vi "UI_HighEnd.vi"() -> ()   [LabVIEW 2021]
uses:
  Common/LabVIEW GEA2 Toolkit/GEA3/type defs/Data Type.ctl
  Controls/All_Bundled_UI.ctl
  Controls/Cluster leds 3-5.ctl
  D:/Common/LabVIEW GEA2 Toolkit/source/GEA3 DLL Source/GeaCommunication.dll
  Common/LabVIEW GEA2 Toolkit/source/GEA3 DLL Source/GeaCommunication.dll
  Common/LabVIEW GEA2 Toolkit/GEA3/library/GEA2_Toolkit.lvlib
panel:
  in  "Cluster Leds 3-5 2":T1
  in  "All_Bundled_UI":T2
  in  "Knob":dbl(knob) scale=0.0..10.0
  in  "PLANCHA FÁCIL":bool caption="PLANCHA\nFÁCIL"
  in  "LAVADO RÁPIDO":bool caption="LAVADO\nRÁPIDO"
  in  "INICIO PAUSA":bool caption="INICIO\nPAUSA"
  in  "VEL CENTRIF.":bool caption="VEL\nCENTRIF."
  in  "INICIO DIFERIDO":bool caption="INICIO\nDIFERIDO"
  in  "SUPER  ENJUAGUE":bool caption="SUPER \nENJUAGUE"
  in  "TEMP.":bool
  out "ERD Data Out":cluster{"ERD Number":u16, "Data":string}[](array[cluster]) {"ERD Number" format="%.0x"}
  in  "Read ERD List":cluster{"ERD Number":u16, "Data Type":T3}[](array[cluster]) {"ERD Number" format="%.0x"}
  in  "GEA Inputs":cluster{"Source":u8, "Destination":u8}={"Source"=229, "Destination"=192} {"Destination" format="%.0x"; "Source" format="%.0x"}
  in  "Read":bool=TRUE
  in  "Stop Button":bool
  # "70°C"
  # "60°C"
  # "40°C"
  # "30°C"
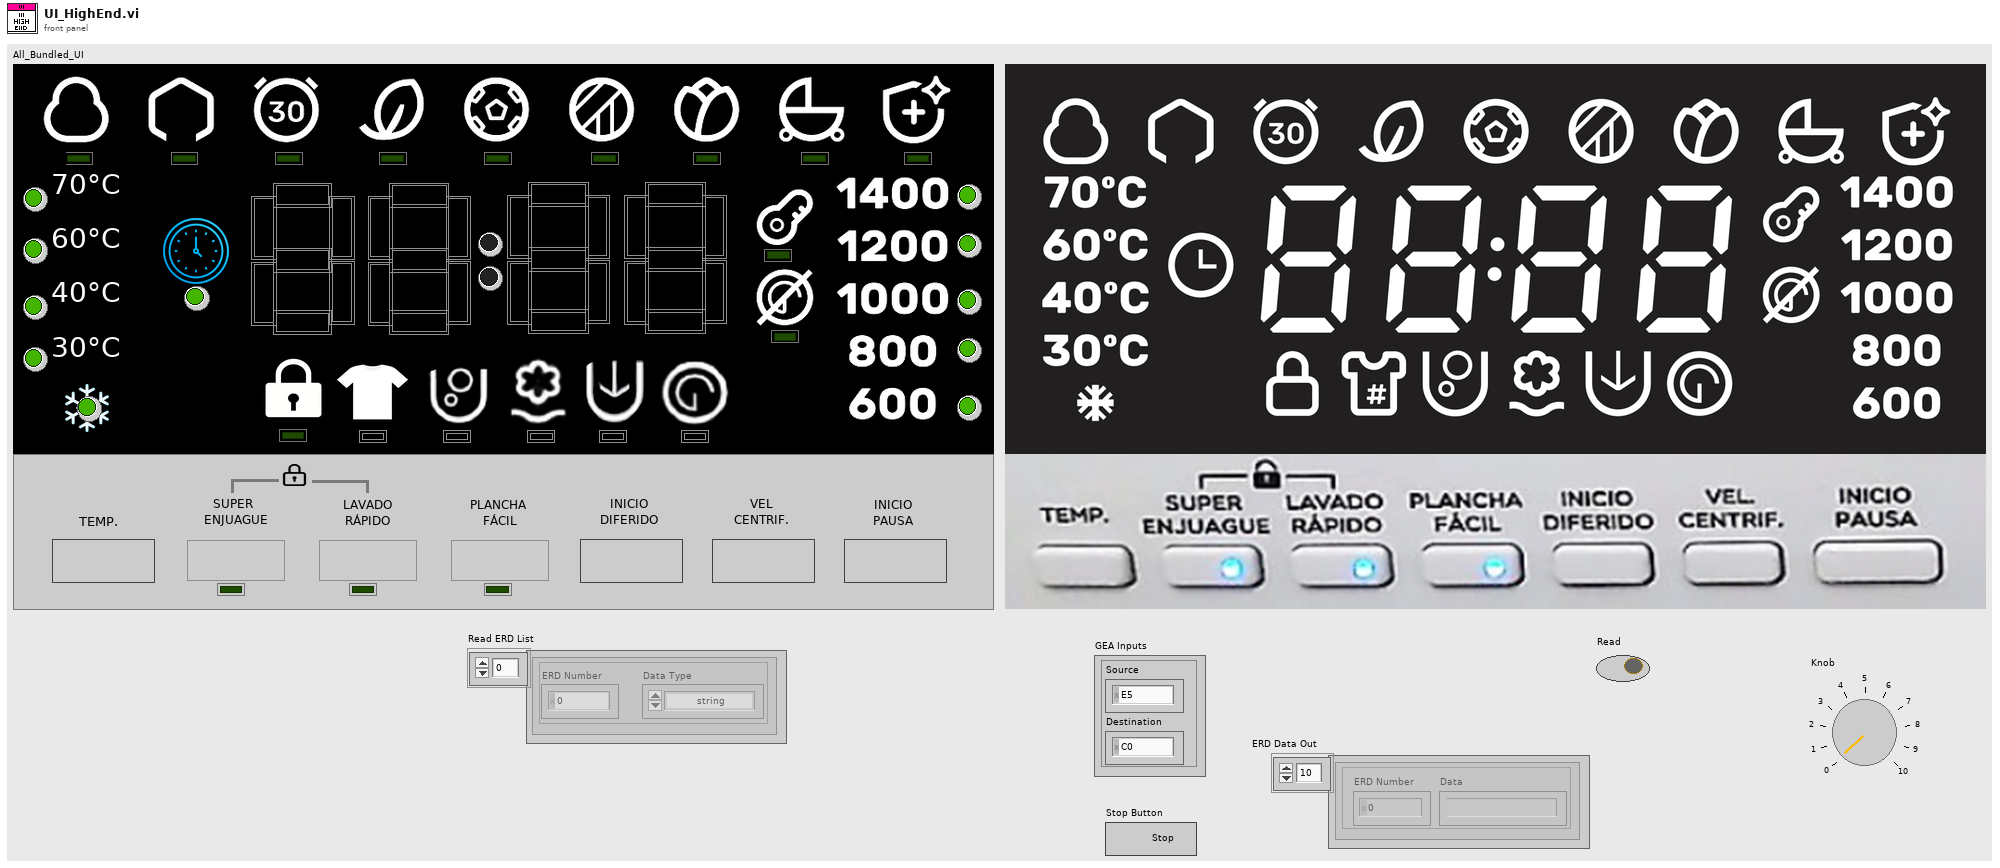
[diagram p1: front panel]
types:
  T1 = typedef "Cluster leds 3-5.ctl" = cluster{"Led03":bool, "Led04":bool, "Led05":bool}
  T2 = typedef "All_Bundled_UI.ctl" = cluster{"Temperature cluster":cluster{"Led nieve":bool, "30°C":bool, "40°C":bool, "60°C":bool, "70°C":bool}, "Cluster Led 11-19":cluster{"Led11":bool, "Led12":bool, "Led13":bool, "Led14":bool, "Led15":bool, "Led16":bool, "Led17":bool, "Led18":bool, "Led19":bool}, "Cluster leds 6-10":cluster{"Led10":bool, "Led09":bool, "Led08":bool, "Led07":bool, "Led06":bool}, "Cluster Icons":cluster{"Iconclock_00":bool, "IconCandado_01":bool, "Icon03":bool, "Icon02":bool}, "Cluster Rpm_level":cluster{"Rpm_level0":bool, "Rpm_level1":bool, "Rpm_level2":bool, "Rpm_level3":bool, "Rpm_level4":bool}, "Display cluster":cluster{"Punto Abajo":bool, "punto Arriba":bool, "Display Millar":cluster{"g4":bool, "f4":bool, "e4":bool, "d4":bool, "c4":bool, "b4":bool, "a4":bool}, "Display Centenas":cluster{"g3":bool, "f3":bool, "e3":bool, "d3":bool, "c3":bool, "b3":bool, "a3":bool}, "Display Decenas":cluster{"g2":bool, "f2":bool, "e2":bool, "d2":bool, "c2":bool, "b2":bool, "a2":bool}, "Display Unidades":cluster{"g1":bool, "f1":bool, "e1":bool, "d1":bool, "c1":bool, "b1":bool, "a1":bool}}}
  T3 = typedef "Data Type.ctl" = enum16{"string", "boolean", "uint8_t", "uint16_t", "uint32_t", "uint64_t", "int8_t", "int16_t", "int32_t", "int64_t"}
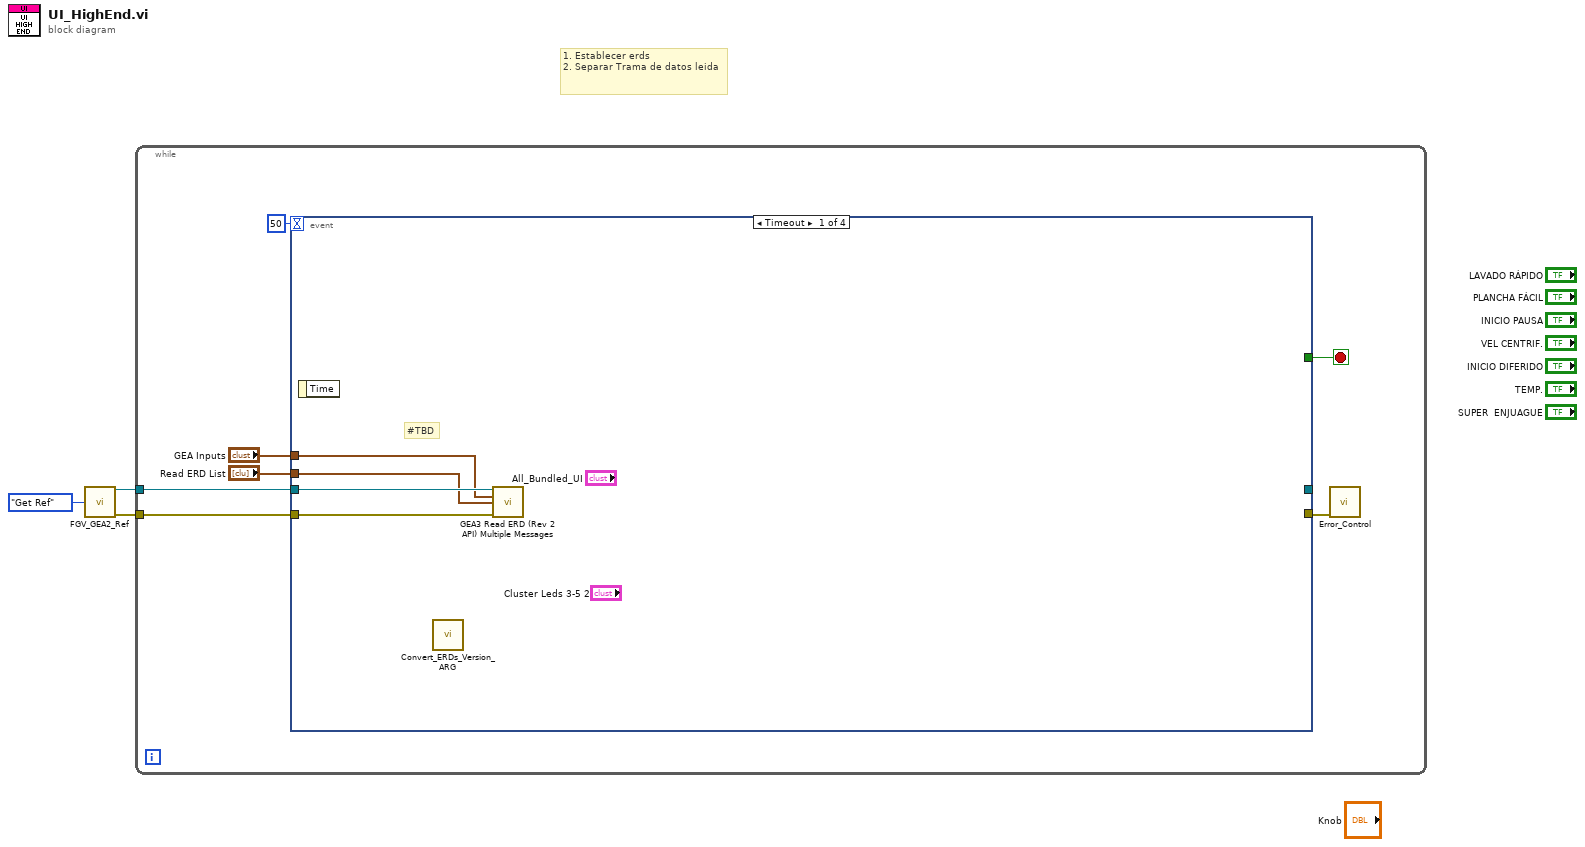
[diagram p0: block diagram]
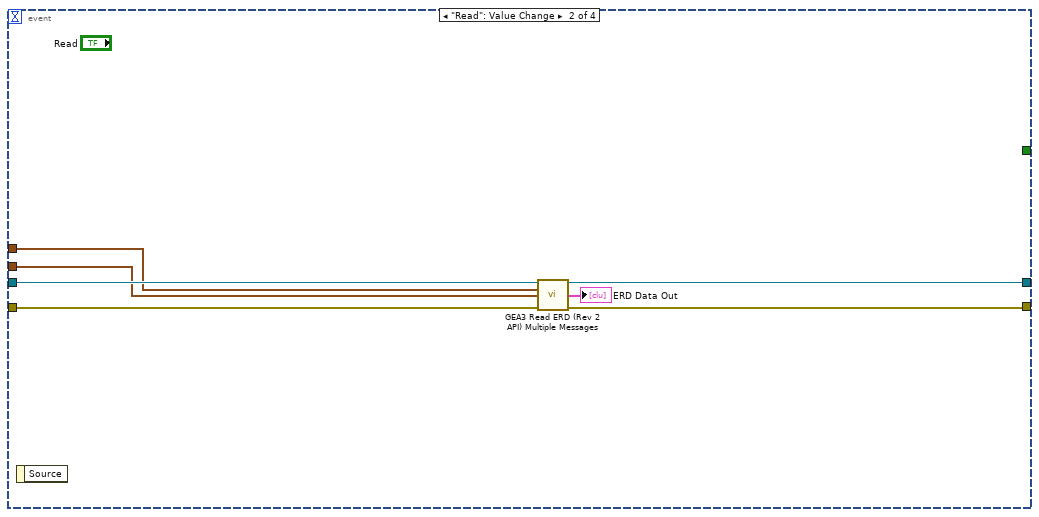
[diagram p2: hidden frame]
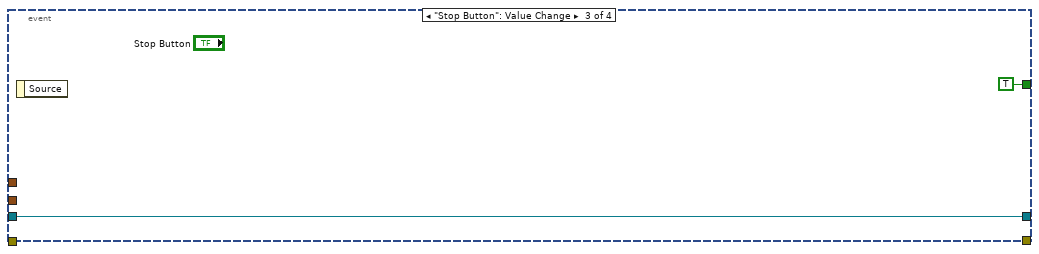
[diagram p3: hidden frame]
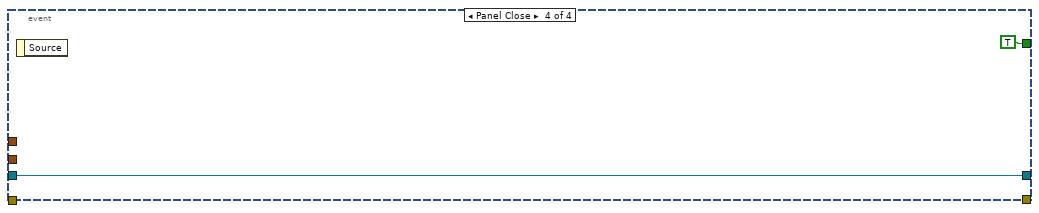
[diagram p4: hidden frame]
diagram:
  # "1. Establecer erds\n2. Separar Trama de datos leida"
  n1 = call "FGV_GEA2_Ref.vi"("Action"=enum16{"Set Ref", "Get Ref"}."Get Ref") -> ("GEA2 Reference Out"=w2:refnum<k24>, "Error Out"=w1:errorcluster)  [unwired: 13 in]
  n2 = while {
    tunnel: w2 -> [w10]
    tunnel: w1 -> [w9]
    stop <- w8 stop-if-true
    n3 = event shown="[0] Timeout" {
      selector: _ -> [_ _ _ _]
      dyn-events: _ -> [_ _ _ _]
      timeout: 50 -> [_ _ _ _]
      tunnel: w10 -> [w14 w21 w22 w24]
      tunnel: w9 -> [w13 w20 _ _]
      tunnel: [_ _ TRUE TRUE] -> w8
      tunnel: "GEA Inputs" -> [w12 w18 _ _]
      tunnel: [_ w17 w22 w24] -> _
      tunnel: [_ w16 _ _] -> w5
      tunnel: "Read ERD List" -> [w11 w15 _ _]
      event Timeout {
        # "#TBD"
        n4 = event-data() -> ()  [unwired: 1 in, 1 out]
        n5 = call "Convert_ERDs_Version_ARG.vi"() -> ()  [unwired: 14 in, 2 out]
        n6 = call "GEA3 Read ERD (Rev 2 API) Multiple Messages.vi"("GEA2 Reference In"=w14, "GEA Inputs"=w12, "Read ERD List"=w11, "Error In"=w13) -> ()  [unwired: 8 in, 4 out]
      }
      event "Read": Value Change {
        n7 = event-data() -> ()  [unwired: 1 in, 1 out]
        n8 = call "GEA3 Read ERD (Rev 2 API) Multiple Messages.vi"("GEA2 Reference In"=w21, "GEA Inputs"=w18, "Read ERD List"=w15, "Error In"=w20) -> ("GEA2 Reference Out"=w17:refnum<k24>, "ERD Data Out"=→"ERD Data Out":cluster{"ERD Number":u16, "Data":string}[], "Error Out"=w16:errorcluster)  [unwired: 8 in, 1 out]
      }
      event "Stop Button": Value Change {
        n9 = event-data() -> ()  [unwired: 1 in, 1 out]
      }
      event Panel Close {
        n10 = event-data() -> ()  [unwired: 1 in, 1 out]
      }
    }
    n11 = call "Error_Control.vi"("Error In"=w5) -> ()  [unwired: 14 in, 1 out]
  }
